vi "ABR-Find Next Level.vi"(0 "Runtime":T1, 11 "error in (no error)":errorcluster) -> (4 "Runtime out":T1, 14 "Finished":bool, 15 "error out":errorcluster)   [LabVIEW 2020]
uses:
  Typedefs/ABR-Runtime Data.ctl
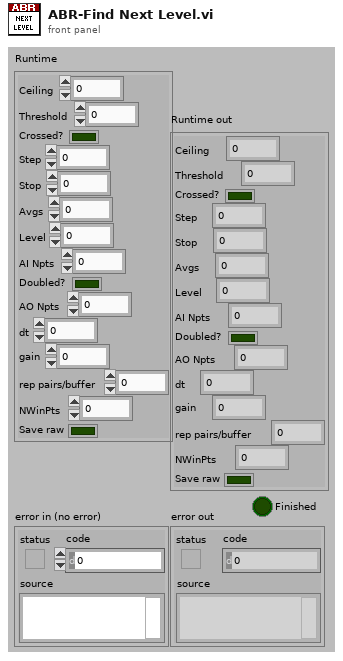
[diagram p1: front panel]
types:
  T1 = typedef "ABR-Runtime Data.ctl" = cluster{"Ceiling":dbl, "Threshold":dbl, "Crossed?":bool, "Step":dbl, "Stop":i32, "Avgs":i32, "Level":dbl, "AI Npts":i32, "Doubled?":bool, "AO Npts":i32, "dt":dbl, "gain":dbl, "rep pairs/buffer":i32, "NWinPts":i32, "Save raw":bool}
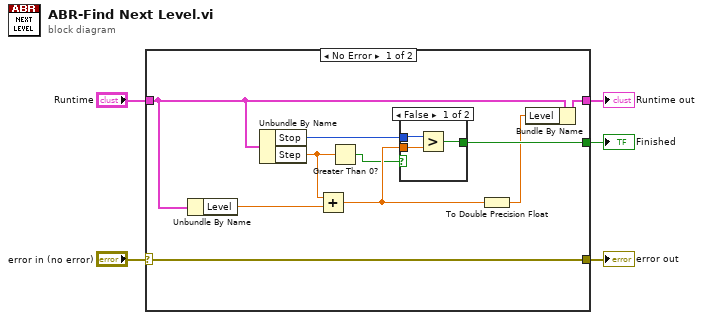
[diagram p0: block diagram]
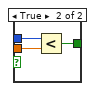
[diagram p2: hidden frame]
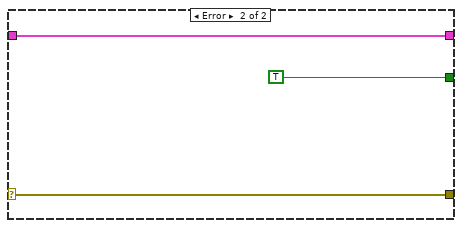
[diagram p3: hidden frame]
diagram:
  n1 = case shown="No Error" "error in (no error)" {
    selector: "error in (no error)" -> [w12 w23]
    tunnel: "Runtime" -> [w8 w24]
    tunnel: [w13 TRUE] -> w3
    tunnel: [w11 w24] -> w2
    tunnel: [w12 w23] -> w1
    frame No Error {
      n2 = Unbundle By Name(w8) -> ("Level"=w9:dbl)
      n3 = Unbundle By Name(w8) -> ("Stop"=w15:i32, "Step"=w7:dbl)
      n4 = Add(x=w7, y=w9) -> (x+y=w14:dbl)
      n5 = Greater Than 0?(x=w7) -> (x > 0?=w6:bool)
      n6 = case shown="False" w6 {
        tunnel: w15 -> [w17 w21]
        tunnel: w14 -> [w16 w20]
        tunnel: [w18 w19] -> w13
        frame False {
          n7 = Greater?(x=w17, y=w16) -> (0:w18:bool)
        }
        frame True {
          n8 = Less?(x=w21, y=w20) -> (x < y?=w19:bool)
        }
      }
      n9 = To Double Precision Float(number=w14) -> (double precision float=w10:dbl)
      n10 = Bundle By Name(cluster=w8, "Level"=w10) -> (w11:T1)
    }
    frame Error {
    }
  }
  "error out" <- w1
  "Runtime out" <- w2
  "Finished" <- w3
